vi "ModelParameterValueSet.vi"(8 "Target":string, 9 "Value":dbl, 10 "Parameter":string) -> (0 "error out":errorcluster, 1 "Target out":string, 2 "Parameter name out":string, 3 "Value out":dbl)   [LabVIEW 2015, in "ni-veristand-steps-runtime-lib.lvlib"]
uses:
  ni-veristand-steps-runtime-lib.lvlib
  <vilib>/NI Veristand/Execution/ModelManager/NI VeriStand - Set Single Parameter Value.vi
  <vilib>/NI Veristand/Execution/ModelManager/NI_VS ModelManager ExecutionAPI.lvlib
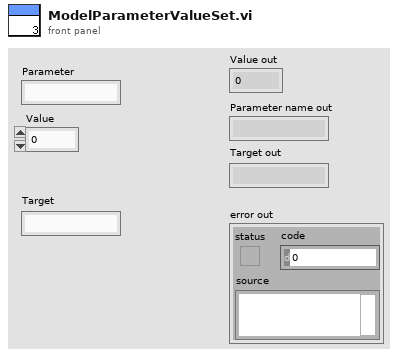
[diagram p1: front panel]
types:
  T1 = typedef "ni-veristand-steps-runtime-lib.lvlib/VeriStand dotNet References.ctl" = cluster{"Project Ref":refnum<k24>, "Workspace Manager Ref":refnum<k24>, "Model Manager Ref":refnum<k24>, "Channel Fault Manager Ref":refnum<k24>}
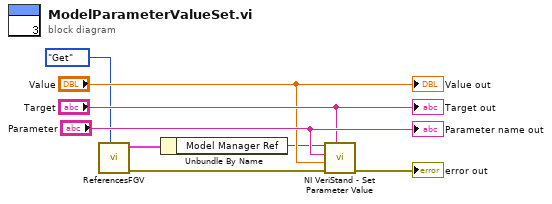
[diagram p0: block diagram]
diagram:
  n1 = call "ReferencesFGV.vi"("Get/Set"=enum16{"Get", "Set"}."Get") -> ("error out"=w3:errorcluster, "VeriStand dotNET Refs out"=w4:T1)  [unwired: 9 in]
  n2 = Unbundle By Name(w4) -> ("Model Manager Ref"=w2:refnum<k24>)
  n3 = call-poly <vilib>:"NI VeriStand - Set Parameter Value.vi"("Target"="Target", "error in (no error)"=w3, "Value"="Value", "Parameter"="Parameter", "ModelManager in"=w2) -> ("error out"=→"error out":errorcluster)  [unwired: 5 in, 1 out]
  "Value out" <- "Value"
  "Parameter name out" <- "Parameter"
  "Target out" <- "Target"
